vi "GetDAQParameter.vi"(2 "Error In":errorcluster) -> (0 "Error Out":errorcluster, 1 "FLIm DAQ":T1)   [LabVIEW 2020]
panel:
  in  "Trigger Delay (s)":dbl format="%#_6p"
  in  "Trigger Level (V)":dbl=0.25 format="%#_6p"
  in  "trigger source":string(combo)="VAL_EXTERNAL"
  in  "Vertical Offset (V)":dbl caption="Vertical Offset"
  in  "Sampling Rate (s/s)":dbl=2.5 format="%.2p"
  in  "Averaging":i32=16
  in  "Timeout (s)":dbl=5.0 format="%.2f"
  in  "Record Length":i32=1000
  in  "Vertical Range (V)":dbl=5.0 format="%.2f"
  in  "Channel(s)":string="0"
  in  "Resource Name":refnum<k15>="PXI1Slot5"
  in  "Confirm":bool
  # "Configuration"
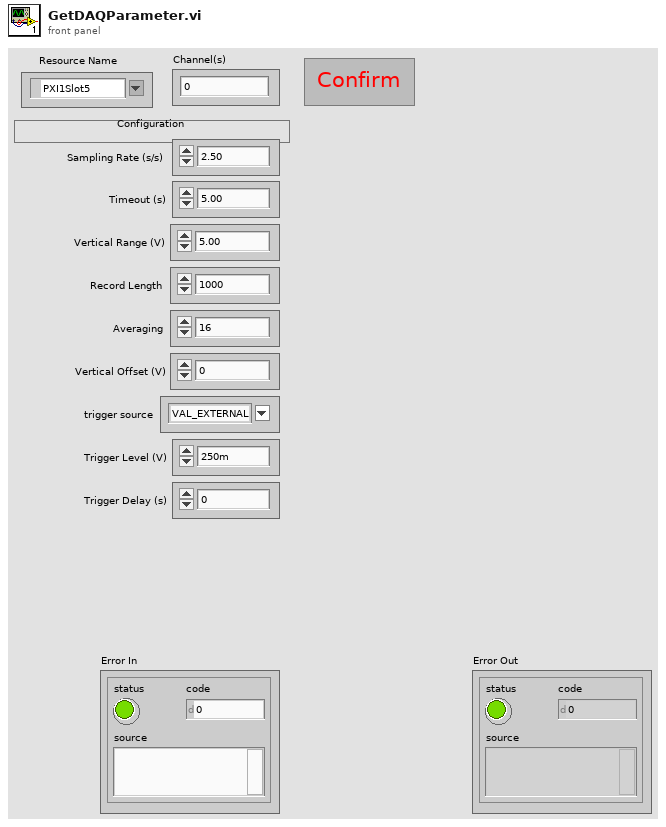
[diagram p1: front panel]
types:
  T1 = cluster{"Resource Name":refnum<k15>, "Channel(s)":string, "Sampling Rate (s/s)":dbl, "Timeout (s)":dbl, "Vertical Range (V)":dbl, "Record Length":i32, "Averaging":i32, "Vertical Offset (V)":dbl, "trigger source":string, "Trigger Level (V)":dbl, "Trigger Delay (s)":dbl}
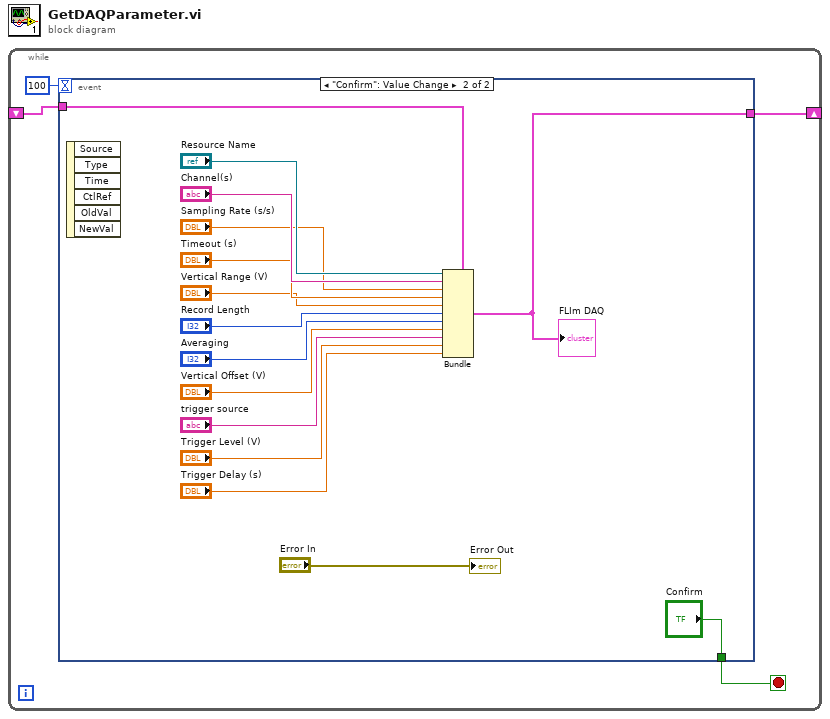
[diagram p0: block diagram]
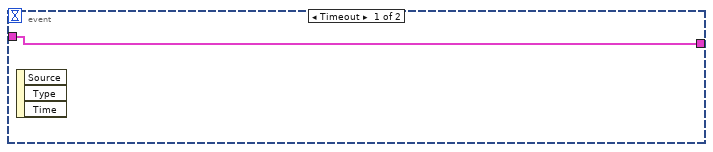
[diagram p2: hidden frame]
diagram:
  n1 = while {
    shift-right: [w2] -> _
    shift-left: _ -> [w3]
    stop <- w1 stop-if-true
    n2 = event shown="[1] \"Confirm\": Value Change" {
      selector: _ -> [_ _]
      dyn-events: _ -> [_ _]
      timeout: 100 -> [_ _]
      tunnel: w3 -> [w5 w7]
      tunnel: [w5 w18] -> w2
      tunnel: [_ "Confirm"] -> w1
      event Timeout {
        n3 = event-data() -> ()  [unwired: 1 in, 3 out]
      }
      event "Confirm": Value Change {
        n4 = event-data() -> ()  [unwired: 1 in, 6 out]
        n5 = Bundle(cluster=w7, "Resource Name"="Resource Name", "Channel(s)"="Channel(s)", "Sampling Rate (s/s)"="Sampling Rate (s/s)", "Timeout (s)"="Timeout (s)", "Vertical Range (V)"="Vertical Range (V)", "Record Length"="Record Length", "Averaging"="Averaging", "Vertical Offset (V)"="Vertical Offset (V)", "trigger source"="trigger source", "Trigger Level (V)"="Trigger Level (V)", "Trigger Delay (s)"="Trigger Delay (s)") -> (w18:T1)
        "FLIm DAQ" <- w18
        "Error Out" <- "Error In"
      }
    }
  }
